vi "Convert I32 to SGL -Virtex5.vi"(0 "Data In":i32, 3 "Data Valid In":bool=TRUE) -> (7 "Data Out":sgl, 10 "Data Valid Out":bool)   [LabVIEW 2014]
uses:
  <vilib>/rvi/IPIntegrationNode/IPINode_Typedef/niFpgaIPINodeSupportedFamilies.ctl
  <vilib>/rvi/IPIntegrationNode/IPINode_Utilities/niFpgaIPINodeSimCore.vi
  <vilib>/rvi/XilinxIP/XIPIN_XNode/niFpgaXIPIN.xnode
  I32toSGL_V5/I32toSGL_V5_5C7CB889465D4178BEAD3C8DDC476BC2.dll
  <vilib>/rvi/IPIntegrationNode/IPINode_Xnode/niFpgaIPINode.xnode
panel:
  # "Copyright 2014 Vidrio Technologies\nScanImage 5 software is licensed under the Apache License, Version 2.0 (the \"License\"); you may not use any files contained\nwithin the ScanImage 5 release except in compliance with the License. You may obtain a copy of the License at\n http://www.apache.org/licenses/LICENSE-2.0\nUnless required by applicable law or agreed to in writing, software distributed under the License is distributed on an\n\"AS IS\" BASIS, WITHOUT WARRANTIES OR CONDITIONS OF ANY KIND, either express or implied. See the License for the\n specific language governing permissions and limitations under the License."
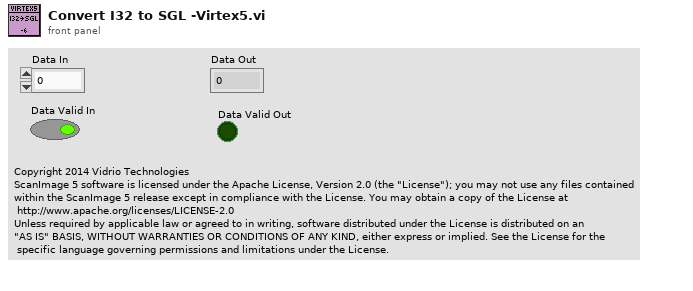
[diagram p1: front panel]
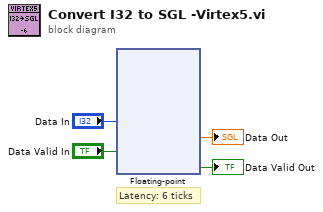
[diagram p0: block diagram]
diagram:
  # "Latency: 6 ticks"
  n1 = xnode ("Floating-point")("a"="Data In", "operation_nd"="Data Valid In") -> ("result"=→"Data Out":sgl, "rdy"=→"Data Valid Out":bool)
